vi "MPP.direction.vi"(8 "error in (no error)":errorcluster, 10 "UP?":bool, 11 "VISA Refnum in":refnum<visa-resource-name>) -> (0 "error out":errorcluster, 3 "VISA Refnum out":refnum<visa-resource-name>)   [LabVIEW 2020, in "main.lvlib"]
uses:
  main.lvlib
  <instrlib>/HH PLA Series/HH PLA Series.lvlib
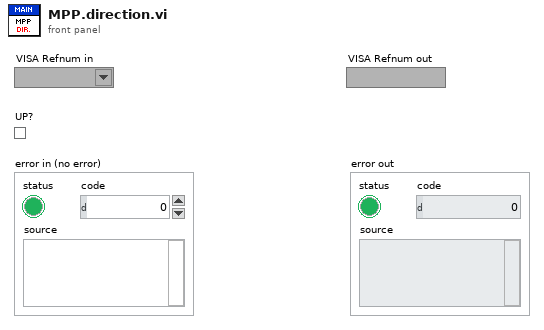
[diagram p1: front panel]
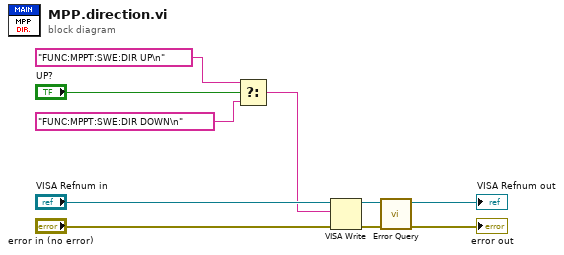
[diagram p0: block diagram]
diagram:
  n1 = Select(t="FUNC:MPPT:SWE:DIR UP\n" ("write buffer"), s="UP?", f="FUNC:MPPT:SWE:DIR DOWN\n" ("write buffer")) -> (s? t:f=w2:string)
  n2 = VISA Write(VISA resource name="VISA Refnum in", write buffer=w2, error in (no error)="error in (no error)") -> (VISA resource name out=w7:refnum<visa-resource-name>, error out=w8:errorcluster)  [unwired: 1 out]
  n3 = call <instrlib>:"Error Query.vi"("error in (no error)"=w8, "VISA resource name"=w7) -> ("error out"=→"error out":errorcluster, "VISA resource name out"=→"VISA Refnum out":refnum<visa-resource-name>)  [unwired: 6 in, 2 out]
